vi "Example 2.vi"   [LabVIEW 2014, in "UI_ProgressDlg.lvlib"]
uses:
  UI_ProgressDlg.lvlib
  _Control/DEF-Type.ctl
  UI_ProgressDlg.lvclass
types:
  T1 = typedef "UI_ProgressDlg.lvlib/UI_ProgressDlg.lvclass/DEF-Type.ctl" = enum16{"Progress Window", "Buzy Window", "Timer Window"}
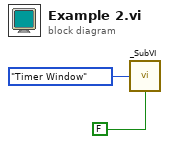
[diagram p0: block diagram]
diagram:
  n1 = call "_SubVI.vi"("Closeable?"=FALSE, "Type"=DEF-Type."Timer Window") -> ()  [unwired: 3 in]
